vi "Shut Down Device.vi"(8 "error in (no error)":errorcluster, 11 "Uniblitz Shutter in":refnum<class "Uniblitz Shutter.lvclass">) -> (0 "error out":errorcluster, 3 "Uniblitz Shutter out":refnum<class "Uniblitz Shutter.lvclass">)   [LabVIEW 2015, in "Uniblitz Shutter.lvlib" / "Uniblitz Shutter.lvclass"]
uses:
  Uniblitz Shutter.lvclass
  <vilib>/DAQmx/write.llb/DAQmx Write (Digital Bool 1Line 1Point).vi
  Device/Device.lvclass
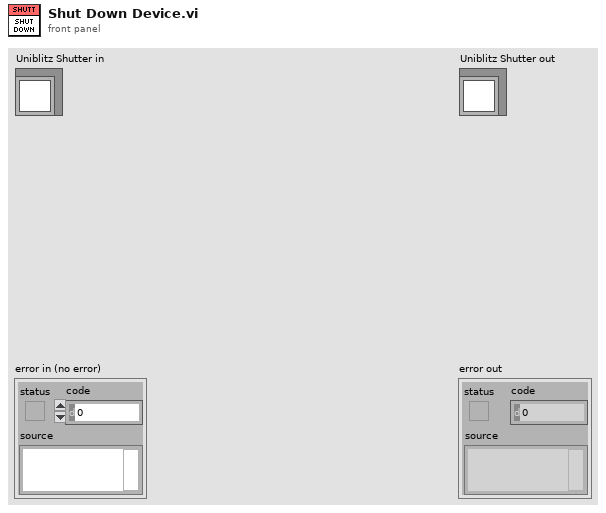
[diagram p1: front panel]
types:
  T1 = typedef "Excitation.ctl" = enum16{"Cy2 (473 nm)", "Cy3 (532 nm)", "Cy5 (639 nm)", "Cy7 (730 nm)"}
  T2 = cluster{"Excitation":T1, "DAQmx Channel":refnum<k21>, "Open?":bool}[]
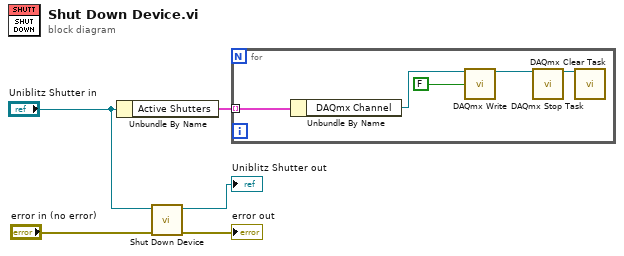
[diagram p0: block diagram]
diagram:
  n1 = Unbundle By Name("Uniblitz Shutter in") -> ("Active Shutters"=w2:T2)
  n2 = call-parent "Shut Down Device.vi"("error in (no error)"="error in (no error)", "Device in"="Uniblitz Shutter in") -> ("error out"=→"error out":errorcluster, "Device out"=→"Uniblitz Shutter out":refnum<class "Uniblitz Shutter.lvclass">)  [unwired: 8 in]
  n3 = for {
    tunnel: w2 -> [w9] mode=indexing
    n4 = Unbundle By Name(w9) -> ("DAQmx Channel"=w7:refnum<k21>)
    n5 = call-poly <vilib>:"DAQmx Write.vi"("task/channels in"=w7, "data"=FALSE) -> ("task out"=w6:refnum<k21>)  [unwired: 11 in, 2 out]
    n6 = call <vilib>:"DAQmx Stop Task.vi"("task/channels in"=w6) -> ("task out"=w10:refnum<k21>)  [unwired: 13 in, 1 out]
    n7 = call <vilib>:"DAQmx Clear Task.vi"("task in"=w10) -> ()  [unwired: 14 in, 1 out]
  }
